vi "ws_about status.vi"(8 "error in (no error)":errorcluster, 11 "Connection Refnum":T1) -> (0 "error out":errorcluster, 3 "keys":T2)   [LabVIEW 2011]
uses:
  <vilib>/addons/internet/utils/keyedarr.llb/Keyed Array.ctl
  SI.LIB/ODBC/SQL Controls/Connection Refnum.ctl
  server/database/Users/User Record.ctl
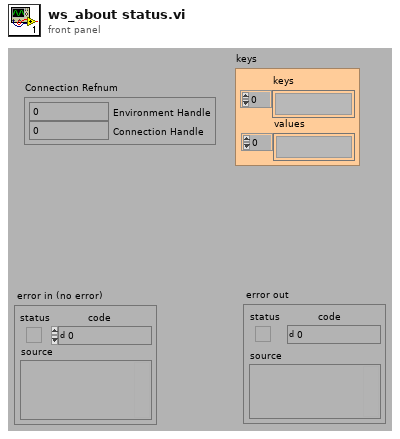
[diagram p1: front panel]
types:
  T1 = typedef "Connection Refnum.ctl" = cluster{"Environment Handle":i32, "Connection Handle":i32}
  T2 = typedef "Keyed Array.ctl" = cluster{"keys":string[], "values":string[]}
  T3 = typedef "User Record.ctl" = cluster{"ixUser":i32, "sxUsername":string, "sLastName":string, "sFirstName":string, "sEmail":string, "sPassword":string, "tLoginTime":timestamp, "sLoginComputer":string, "fAdministrator":bool, "fRunSequences":bool, "fModifySequences":bool, "fRunScenarios":bool, "fModifyScenarios":bool, "fModifyTemplates":bool, "fModifyUsers":bool, "fModifyStations":bool, "fModifyFields":bool}
  T4 = typedef "OGAB Version.ctl" = cluster{"Version":string, "Build Number":u32, "Build Date/Time":dbl}
  T5 = cluster{"Index Size, bytes":i64, "Index Date":dbl, "Test Files":i32, "Test Runs":i32}
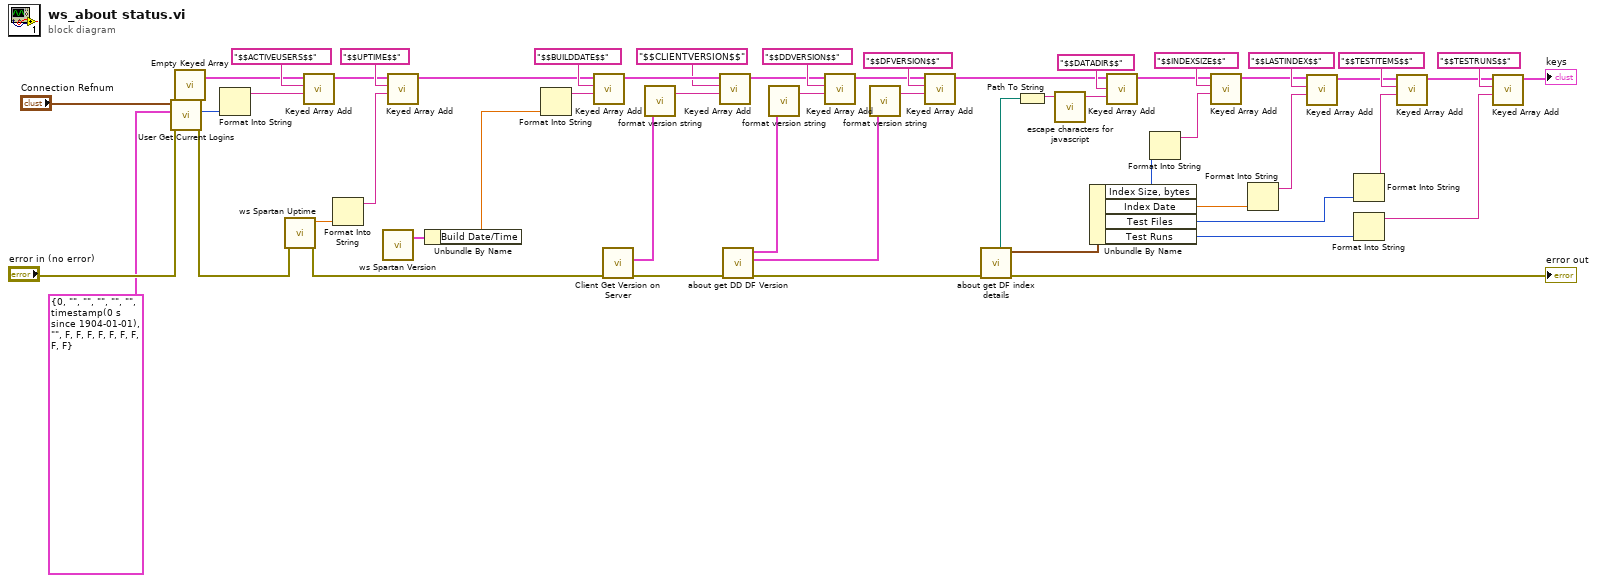
[diagram p0: block diagram]
diagram:
  n1 = call "User Get Current Logins.vi"("error in (no error)"="error in (no error)", "Current User (none)"=T3 {"ixUser"=0, "sxUsername"="", "sLastName"="", "sFirstName"="", "sEmail"="", "sPassword"="", "tLoginTime"=timestamp(0 s since 1904-01-01), "sLoginComputer"="", "fAdministrator"=FALSE, "fRunSequences"=FALSE, "fModifySequences"=FALSE, "fRunScenarios"=FALSE, "fModifyScenarios"=FALSE, "fModifyTemplates"=FALSE, "fModifyUsers"=FALSE, "fModifyStations"=FALSE, "fModifyFields"=FALSE}, "Connection Refnum"="Connection Refnum") -> ("error out"=w9:errorcluster, "Seats in Use"=w14:i32)  [unwired: 7 out]
  n2 = call "Empty Keyed Array.vi"() -> ("empty keyed array"=w16:T2)  [unwired: 3 out]
  n3 = Format Into String(w14) -> (resulting string=w15:string)  [unwired: 3 in, 1 out]
  n4 = call "ws Spartan Uptime.vi"("error in (no error)"=w9) -> ("error out"=w8:errorcluster, "Uptime"=w7:dbl)  [unwired: 9 in]
  n5 = call <vilib>:"Keyed Array Add.vi"("value"=w15, "key"="$$ACTIVEUSERS$$" ("Template (\"\")"), "array in"=w16) -> ("array out"=w17:T2)  [unwired: 1 in, 3 out]
  n6 = Format Into String(w7) -> (resulting string=w19:string)  [unwired: 3 in, 1 out]
  n7 = call "ws Spartan Version.vi"() -> ("Version"=w10:T4)  [unwired: 3 in]
  n8 = call <vilib>:"Keyed Array Add.vi"("value"=w19, "key"="$$UPTIME$$" ("Template (\"\")"), "array in"=w17) -> ("array out"=w21:T2)  [unwired: 1 in, 3 out]
  n9 = Unbundle By Name(w10) -> ("Build Date/Time"=w55:dbl)
  n10 = Format Into String(w55) -> (resulting string=w54:string)  [unwired: 3 in, 1 out]
  n11 = call <vilib>:"Keyed Array Add.vi"("value"=w54, "key"="$$BUILDDATE$$" ("Template (\"\")"), "array in"=w21) -> ("array out"=w53:T2)  [unwired: 1 in, 3 out]
  n12 = call "Client Get Version on Server.vi"("error in (no error)"=w8) -> ("error out"=w36:errorcluster, "Version"=w42:T4)  [unwired: 9 out]
  n13 = call "format version string.vi"("Version"=w42) -> ("Version String"=w41:string)  [unwired: 2 out]
  n14 = call <vilib>:"Keyed Array Add.vi"("value"=w41, "key"="$$CLIENTVERSION$$" ("Template (\"\")"), "array in"=w53) -> ("array out"=w50:T2)  [unwired: 1 in, 3 out]
  n15 = call "about get DD DF Version.vi"("error in (no error)"=w36) -> ("error out"=w35:errorcluster, "DF Version"=w32:T4, "DD Version"=w34:T4)  [unwired: 8 out]
  n16 = call "format version string.vi"("Version"=w34) -> ("Version String"=w33:string)  [unwired: 2 out]
  n17 = call <vilib>:"Keyed Array Add.vi"("value"=w33, "key"="$$DDVERSION$$" ("Template (\"\")"), "array in"=w50) -> ("array out"=w48:T2)  [unwired: 1 in, 3 out]
  n18 = call "format version string.vi"("Version"=w32) -> ("Version String"=w31:string)  [unwired: 2 out]
  n19 = call <vilib>:"Keyed Array Add.vi"("value"=w31, "key"="$$DFVERSION$$" ("Template (\"\")"), "array in"=w48) -> ("array out"=w5:T2)  [unwired: 1 in, 3 out]
  n20 = call "about get DF index details.vi"("error in (no error)"=w35) -> ("error out"=→"error out":errorcluster, "Index Details"=w28:T5, "Data Repository Path"=w3:path)  [unwired: 8 out]
  n21 = Path To String(path=w3) -> (string=w2:string)
  n22 = call "escape characters for javascript.vi"("String (\"\")"=w2) -> ("escaped String"=w1:string)  [unwired: 4 in]
  n23 = Unbundle By Name(w28) -> ("Index Size, bytes"=w27:i64, "Index Date"=w26:dbl, "Test Files"=w25:i32, "Test Runs"=w24:i32)
  n24 = call <vilib>:"Keyed Array Add.vi"("value"=w1, "key"="$$DATADIR$$" ("Template (\"\")"), "array in"=w5) -> ("array out"=w4:T2)  [unwired: 1 in, 3 out]
  n25 = Format Into String(w27) -> (resulting string=w40:string)  [unwired: 3 in, 1 out]
  n26 = call <vilib>:"Keyed Array Add.vi"("value"=w40, "key"="$$INDEXSIZE$$" ("Template (\"\")"), "array in"=w4) -> ("array out"=w30:T2)  [unwired: 1 in, 3 out]
  n27 = Format Into String(w26) -> (resulting string=w37:string)  [unwired: 3 in, 1 out]
  n28 = call <vilib>:"Keyed Array Add.vi"("value"=w37, "key"="$$LASTINDEX$$" ("Template (\"\")"), "array in"=w30) -> ("array out"=w29:T2)  [unwired: 1 in, 3 out]
  n29 = Format Into String(w25) -> (resulting string=w39:string)  [unwired: 3 in, 1 out]
  n30 = Format Into String(w24) -> (resulting string=w38:string)  [unwired: 3 in, 1 out]
  n31 = call <vilib>:"Keyed Array Add.vi"("value"=w39, "key"="$$TESTITEMS$$" ("Template (\"\")"), "array in"=w29) -> ("array out"=w43:T2)  [unwired: 1 in, 3 out]
  n32 = call <vilib>:"Keyed Array Add.vi"("value"=w38, "key"="$$TESTRUNS$$" ("Template (\"\")"), "array in"=w43) -> ("array out"=→"keys":T2)  [unwired: 1 in, 3 out]
